vi "Command_Drive_Distance.vi"(0 "Startup":bool, 2 "Distance":dbl, 3 "Timeout":dbl=3.0) -> (5 "Reinit":bool, 6 "Completed":bool=TRUE, 7 "Speeds":dbl[](array[numeric]))   [LabVIEW 2018]
uses:
  Global_Variables/Sensor_Values.vi
panel:
  in  "kP_Turn":dbl=-0.038
  in  "kP":dbl=0.005
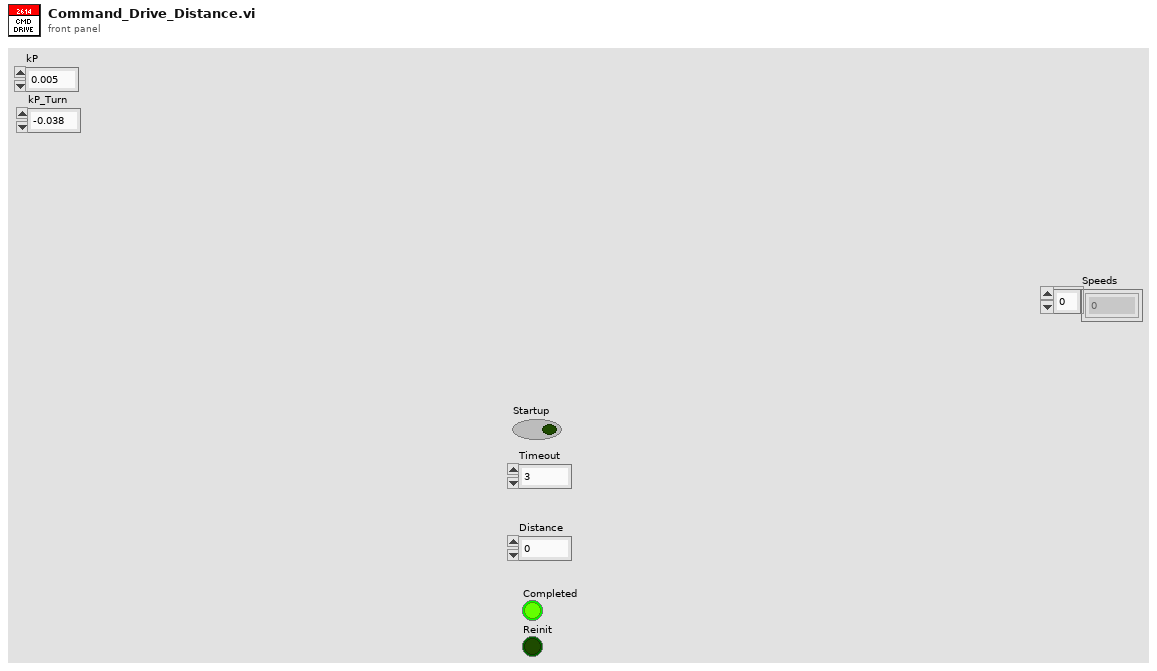
[diagram p1: front panel]
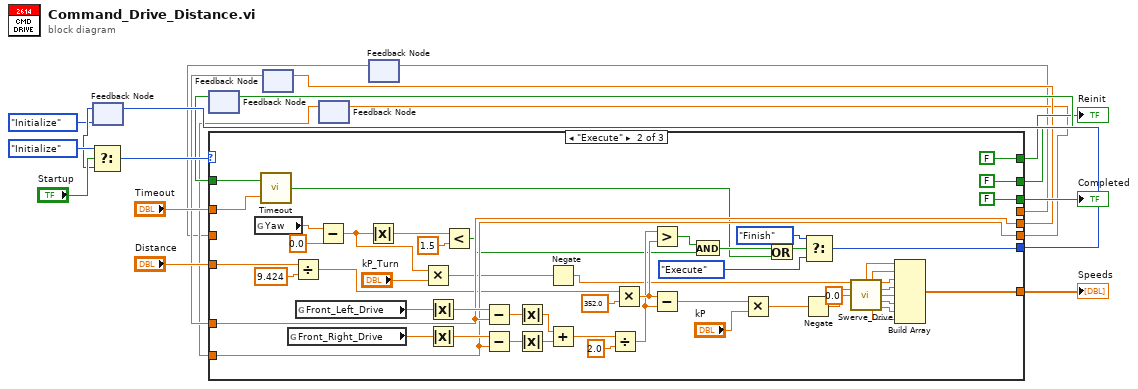
[diagram p0: block diagram]
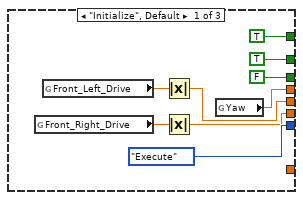
[diagram p2: hidden frame]
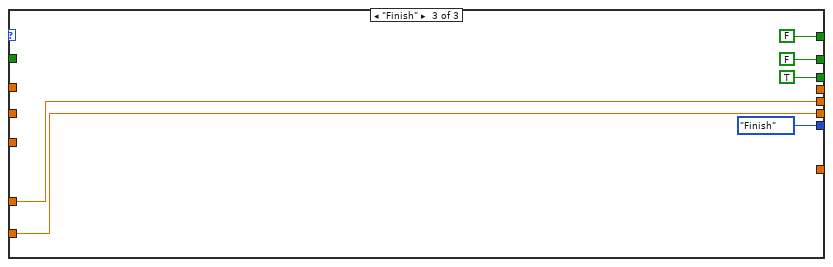
[diagram p3: hidden frame]
diagram:
  n1 = feedback #1(enum16{"Initialize", "Execute", "Finish"}."Initialize" ("f")) -> (w15:enum16{"Initialize", "Execute", "Finish"})
  n2 = Select(t=enum16{"Initialize", "Execute", "Finish"}."Initialize", s="Startup", f=w15) -> (s? t:f=w19:enum16{"Initialize", "Execute", "Finish"})
  n3 = feedback #2() -> (w13:bool)  [unwired: 1 in]
  n4 = feedback #3() -> (w6:dbl)  [unwired: 1 in]
  n5 = feedback #4() -> (w3:dbl)  [unwired: 1 in]
  n6 = feedback #5() -> (w1:dbl)  [unwired: 1 in]
  n7 = case shown="\"Execute\"" w19 {
    tunnel: [enum16{"Initialize", "Execute", "Finish"}."Execute" w78 enum16{"Initialize", "Execute", "Finish"}."Finish" ("f")] -> w16
    tunnel: w13 -> [_ w76 _]
    tunnel: [TRUE FALSE FALSE] -> w14
    tunnel: [FALSE FALSE TRUE] -> w12
    tunnel: [TRUE FALSE FALSE] -> w11
    tunnel: "Timeout" -> [_ w73 _]
    tunnel: "Distance" -> [_ w50 _]
    tunnel: w6 -> [_ w69 w83]
    tunnel: [w23 w69 w83] -> w7
    tunnel: [_ w60 _] -> w5
    tunnel: [w21 w56 w82] -> w4
    tunnel: w3 -> [_ w56 w82]
    tunnel: w1 -> [_ _ _]
    tunnel: [w20 _ _] -> w2
    frame "Initialize", Default {
      n8 = global read "Sensor_Values.vi" "Front_Right_Drive"() -> (w22:dbl)
      n9 = global read "Sensor_Values.vi" "Front_Left_Drive"() -> (w24:dbl)
      n10 = Absolute Value(x=w24) -> (abs(x)=w23:dbl)
      n11 = Absolute Value(x=w22) -> (abs(x)=w21:dbl)
      n12 = global read "Sensor_Values.vi" "Yaw"() -> (w20:dbl)
    }
    frame "Execute" {
      n13 = global read "Sensor_Values.vi" "Yaw"() -> (w38:dbl)
      n14 = call "Timeout.vi"("Timeout"=w73, "Initialize"=w76) -> ("Timed Out?"=w30:bool)
      n15 = global read "Sensor_Values.vi" "Front_Right_Drive"() -> (w58:dbl)
      n16 = Divide(x=w50, y=9.424) -> (x/y=w48:dbl)
      n17 = global read "Sensor_Values.vi" "Front_Left_Drive"() -> (w72:dbl)
      n18 = Subtract(x=w38, y=0.0) -> (x-y=w34:dbl)
      n19 = Absolute Value(x=w34) -> (abs(x)=w36:dbl)
      n20 = Multiply(x=w34, y="kP_Turn") -> (x*y=w41:dbl)
      n21 = Absolute Value(x=w72) -> (abs(x)=w71:dbl)
      n22 = Absolute Value(x=w58) -> (abs(x)=w57:dbl)
      n23 = Less?(x=w36, y=1.5) -> (x < y?=w32:bool)
      n24 = Subtract(x=w71, y=w69) -> (x-y=w70:dbl)
      n25 = Subtract(x=w57, y=w56) -> (x-y=w59:dbl)
      n26 = Absolute Value(x=w70) -> (abs(x)=w55:dbl)
      n27 = Absolute Value(x=w59) -> (abs(x)=w54:dbl)
      n28 = Negate(x=w41) -> (-x=w37:dbl)
      n29 = Add(x=w55, y=w54) -> (x+y=w53:dbl)
      n30 = Divide(x=w53, y=2.0) -> (x/y=w45:dbl)
      n31 = Multiply(x=w48, y=352.0) -> (x*y=w46:dbl)
      n32 = Greater?(x=w45, y=w46) -> (0:w51:bool)
      n33 = Subtract(x=w46, y=w45) -> (x-y=w40:dbl)
      n34 = And(x=w51, y=w32) -> (x .and. y?=w74:bool)
      n35 = Multiply(x=w40, y="kP") -> (x*y=w44:dbl)
      n36 = Or(x=w74, y=w30) -> (x .or. y?=w31:bool)
      n37 = Negate(x=w44) -> (-x=w42:dbl)
      n38 = Select(t=enum16{"Initialize", "Execute", "Finish"}."Finish", s=w31, f=enum16{"Initialize", "Execute", "Finish"}."Execute") -> (s? t:f=w78:enum16{"Initialize", "Execute", "Finish"})
      n39 = call "Swerve_Drive.vi"("Z"=w37, "Y"=w42, "X"=0.0) -> ("Back Left Spin Speed"=w68:dbl, "Back Right Spin Speed"=w67:dbl, "Front Left Spin Speed"=w66:dbl, "Front Right Spin Speed"=w65:dbl, "Back Left Motor Power"=w64:dbl, "Back Right Motor Power"=w63:dbl, "Front Right Motor Power"=w61:dbl, "Front Left Motor Power"=w62:dbl)  [unwired: 5 in]
      n40 = Build Array(w68, w67, w66, w65, w64, w63, w62, w61) -> (w60:dbl[])
    }
    frame "Finish" {
    }
  }
  "Completed" <- w12
  "Reinit" <- w11
  "Speeds" <- w5
  n41 = feedback-in #1(w16) -> ()
  n42 = feedback-in #2(w14) -> ()
  n43 = feedback-in #3(w7) -> ()
  n44 = feedback-in #4(w4) -> ()
  n45 = feedback-in #5(w2) -> ()
